vi "Split Lines.vi"(8 "error in":errorcluster, 10 "String Camera Status":string, 11 "Construct String Camera Status in":refnum<class "Construct String Camera Status.lvclass">) -> (0 "error out":errorcluster, 2 "array":string[](array[string]), 3 "Construct String Camera Status out":refnum<class "Construct String Camera Status.lvclass">)   [LabVIEW 2018, in "Construct String Camera Status.lvclass"]
doc: "Este VI recebe uma string, retornando um array onde cada elemento é uma das linhas da string."
uses:
  Construct String Camera Status.lvclass
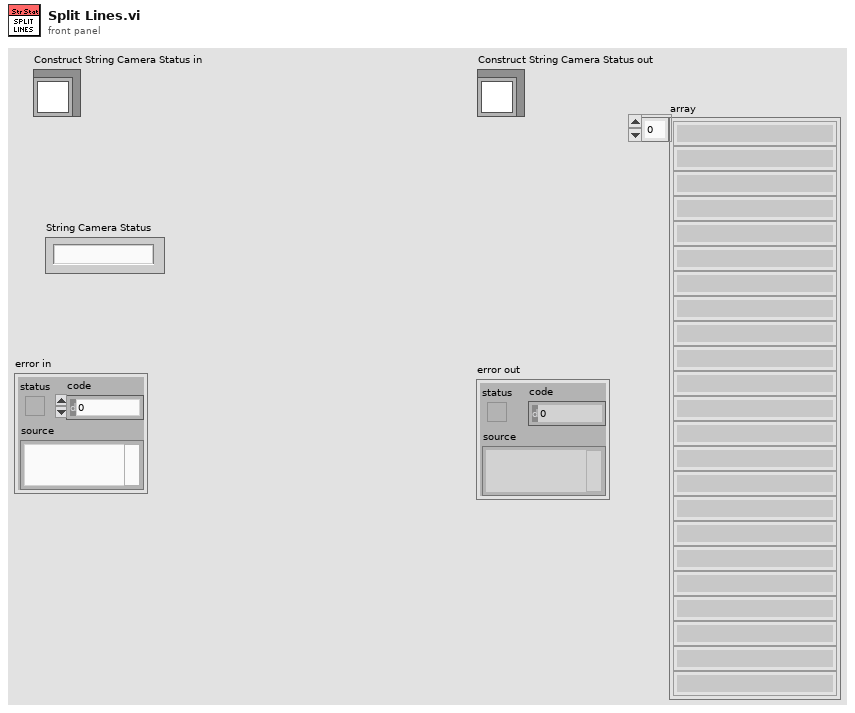
[diagram p1: front panel]
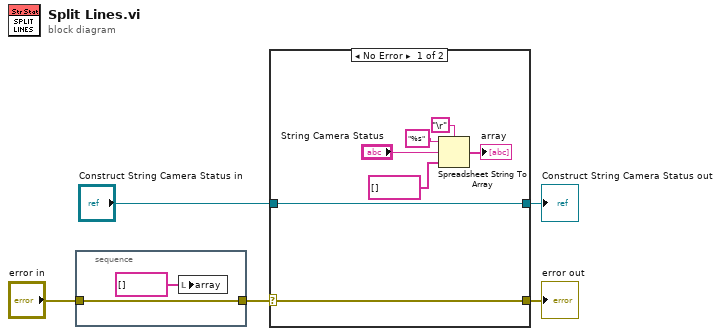
[diagram p0: block diagram]
diagram:
  n1 = stacked-sequence {
    tunnel: "error in" -> [w6]
    tunnel: [w6] -> w2
    frame #0 {
      n2 = local write "array"(string[] []) -> ()
    }
  }
  n3 = case shown="No Error" w2 {
    selector: w2 -> [w14 w15]
    tunnel: [w14 w15] -> w5
    tunnel: [w13 w16] -> w3
    tunnel: "Construct String Camera Status in" -> [w13 w16]
    frame No Error {
      n4 = Spreadsheet String To Array(delimiter (Tab)="\r", format string="%s", spreadsheet string="String Camera Status", array type (2D Dbl)=string[] []) -> (array=→"array":string[])
    }
    frame Error {
    }
  }
  "error out" <- w5
  "Construct String Camera Status out" <- w3
